vi "Bertta_v06_1.vi"() -> ()   [LabVIEW 2015]
uses:
  BERTTA.dll
panel:
  in  "Tab Control":T1(tab)
  in  "Description":string
  in  "Project name":string
  in  "User (initials)":string
  out "Tr":dbl
  out "Tj":dbl
  out "Numeric 2":dbl
  out "Numeric 3":dbl
  out "Numeric":dbl
  out "Mettler 5":dynamicdata(graph)
  out "Temp":dynamicdata(graph)
  out "Mettler":dynamicdata(graph)
  in  "Balances":bool[](array[boolean])
  out "Waveform Chart 3":dynamicdata(graph)
  out "Table":string[][](table)
  in  "Headers":string[](array[string])
  in  "?":bool
  in  "Seq":dbl[][](array[numeric])=[[20.0, 60.0, 40.0], [60.0, 40.0, 20.0], [100.0, 100.0, 100.0]]
  out "Elapsed":i32
  out "Step":i32
  out "Sp":dbl
  out "T":dbl
  out "Tinit":dbl
  out "Tset":dbl
  out "Time constant":dbl
  out "Sp - Tset":i32
  out "Change":i32
  out "Waveform Chart":dynamicdata(graph)
  in  "Tbypass":dbl=33.0
  in  "Tfail":dbl=22.0
  in  "err":i32
  in  "PAUSE":bool
  out "Waveform Chart 2":dynamicdata(graph)
  out "Rate (g/s)":dbl
  out "Time (s)":dbl
  out "Target (g)":dbl
  in  "Seq 2":dbl[][](array[numeric])=[[20.0, 60.0, 40.0], [60.0, 40.0, 20.0], [100.0, 100.0, 100.0]]
  out "Weight (1)":dbl
  out "target reached":i32
  out "x/y":dbl
  out "bal_previous":i32
  out "Step":i32
  in  "?":bool
  in  "Bypass ramp":dbl
  in  "bypass 2":bool
  out "DAQ assistant (4-20 mA)":dbl
  out "Step":i32
  out "bal_previous":i32
  out "x/y":dbl
  out "target reached":i32
  out "Waveform Chart 5":dynamicdata(graph)
  out "Weight (2)":dbl
  out "Rate (g/s)":dbl
  out "Time (s)":dbl
  out "Target (g)":dbl
  in  "Seq 3":dbl[][](array[numeric])=[[20.0, 60.0, 40.0], [60.0, 40.0, 20.0], [100.0, 100.0, 100.0]]
  in  "Boolean":bool
  in  "Bypass ramp":dbl
  in  "bypass":bool
  out "RS232 to Ismatec":dbl
  in  "Boolean 2":bool
  out "Step":i32
  out "bal_previous":i32
  out "x/y":dbl
  out "target reached":i32
  out "Waveform Chart 6":dynamicdata(graph)
  out "Weight (3)":dbl
  out "Rate (g/s)":dbl
  out "Time (s)":dbl
  out "Target (g)":dbl
  in  "Seq 4":dbl[][](array[numeric])=[[20.0, 60.0, 40.0], [60.0, 40.0, 20.0], [100.0, 100.0, 100.0]]
  in  "Boolean 3":bool
  out "Step":i32
  out "bal_previous":i32
  out "x/y":dbl
  out "target reached":i32
  out "Waveform Chart 7":dynamicdata(graph)
  out "Weight (4)":dbl
  out "Rate (g/s)":dbl
  out "Time (s)":dbl
  out "Target (g)":dbl
  in  "Seq 5":dbl[][](array[numeric])=[[20.0, 60.0, 40.0], [60.0, 40.0, 20.0], [100.0, 100.0, 100.0]]
  out "RPM":dbl
  out "Waveform Chart 4":dynamicdata(graph)
  in  "Set RPM":dbl(slide) scale=0.0..500.0
  out "Torque":dbl
  in  "?":T2(tab)
  in  "Device port":dbl=1.0
  out "Debug msg":dbl
  in  "Device port":dbl=8.0
  in  "Device port":i32=2
  in  "Device port 2":i32=6
  in  "Device port 3":i32=7
  in  "Device port 4":i32=10
  # "1"
  # "2"
  # "3"
  # "4"
  # "Step 1"
  # "Step 2"
  # "Step 3"
  # "Step 4"
  # "Step 1"
  # "Step 2"
  # "Step 3"
  # "Step 4"
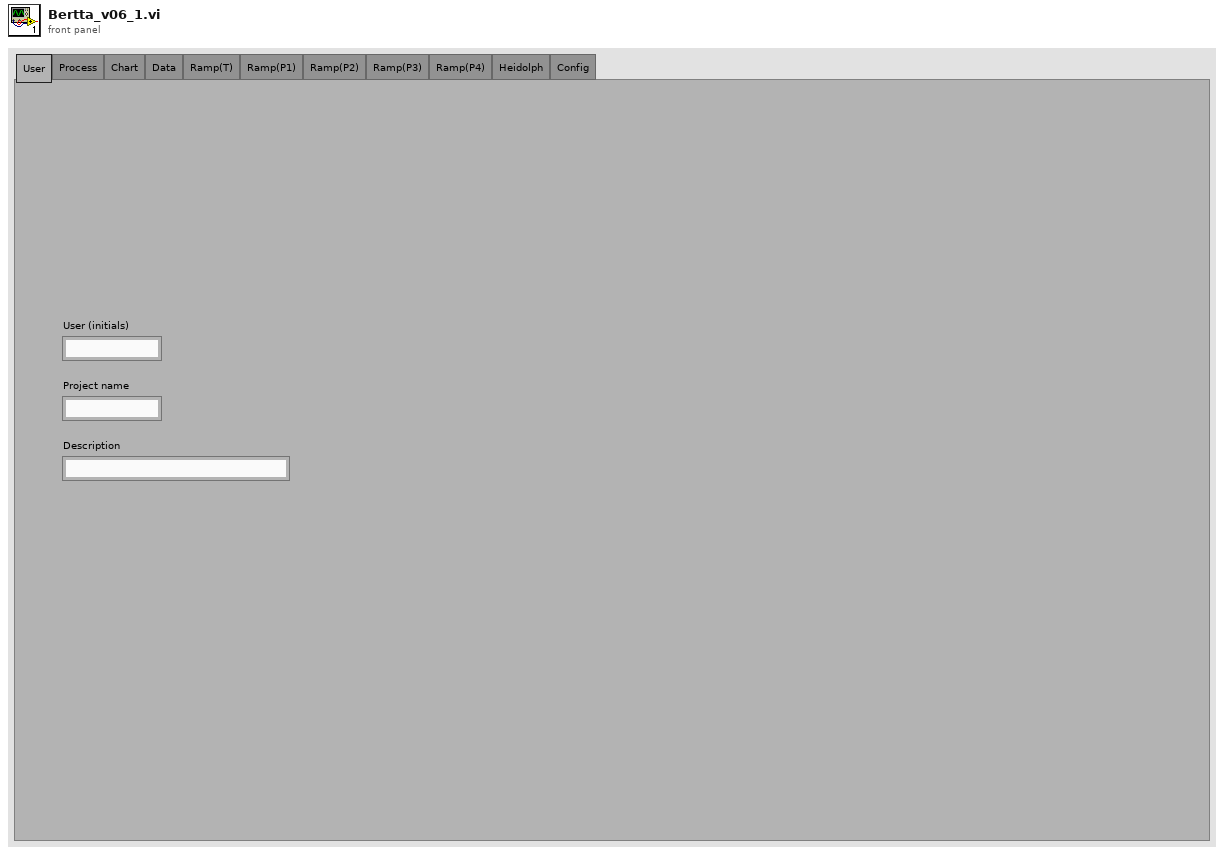
[diagram p1: front panel]
types:
  T1 = enum32{"User", "Process", "Chart", "Data", "Ramp(T)", "Ramp(P1)", "Ramp(P2)", "Ramp(P3)", "Ramp(P4)", "Heidolph", "Config"}
  T2 = enum32{"DB / File", "Lauda", "Heidolph", "Mettler 1", "Mettler 2", "Mettler 3", "Ismatec 1"}
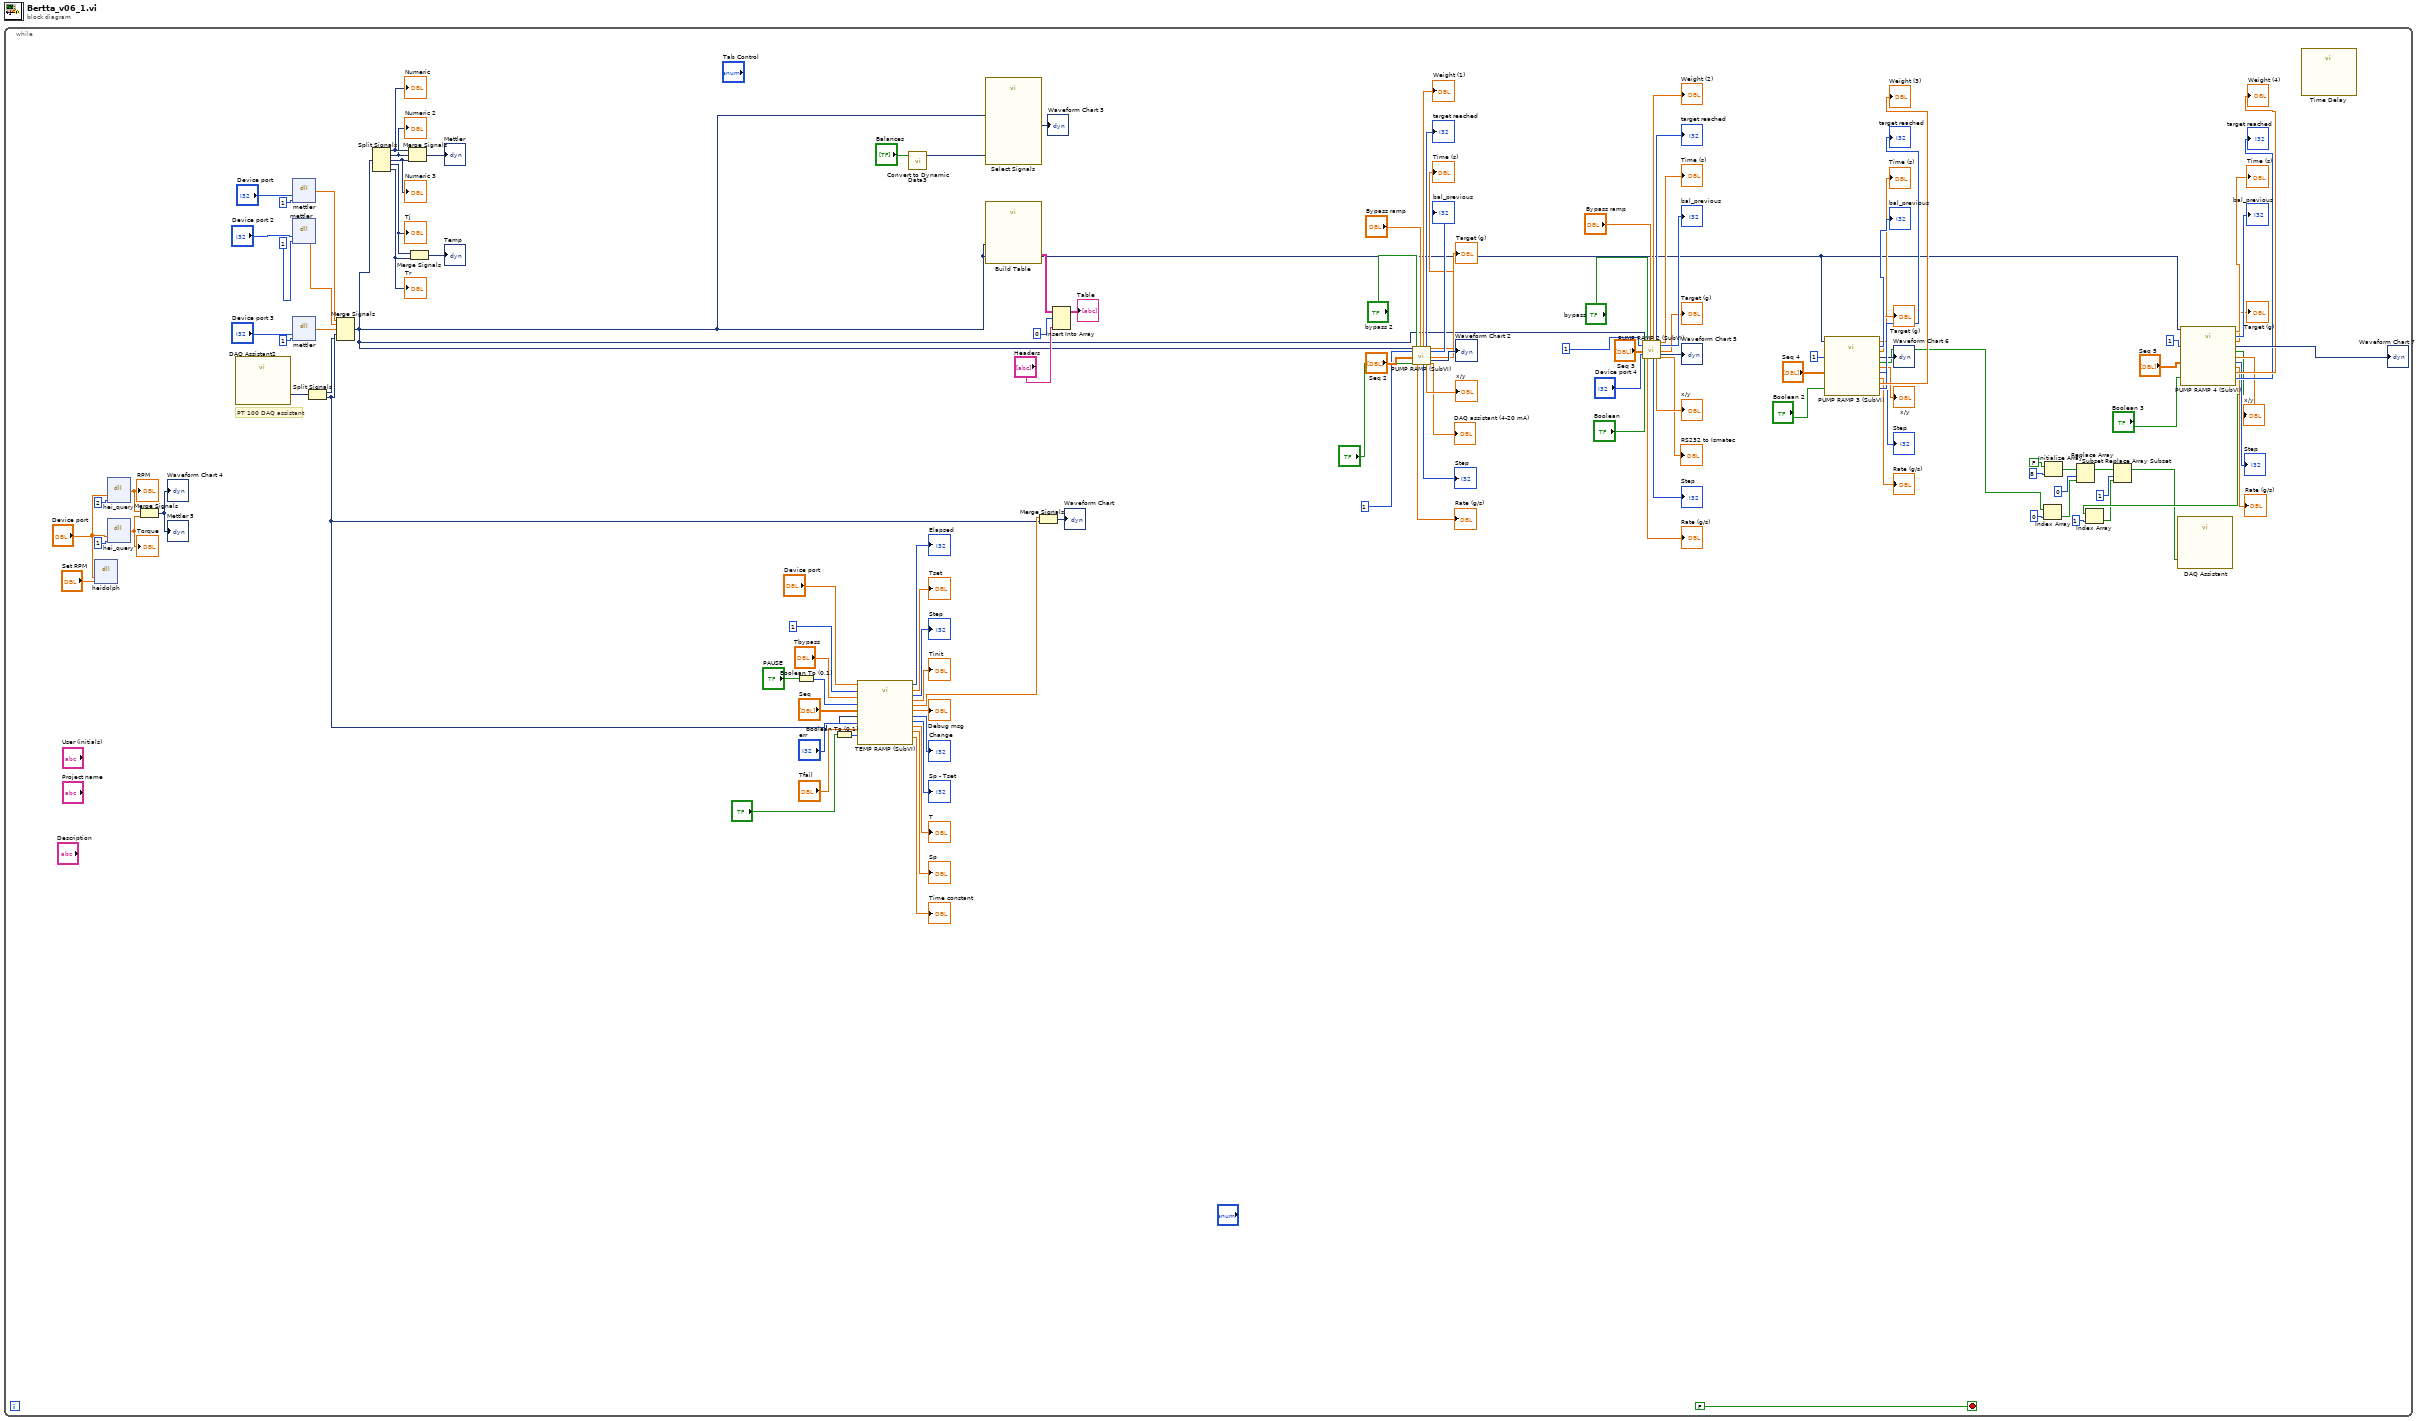
[diagram p0: block diagram]
diagram:
  n1 = while {
    stop <- FALSE stop-if-true
    # "PT 100 DAQ assistant"
    n2 = dll-call lib="C:/Users/xlaraser/Documents/Visual Studio 2017/Projects/Bertta/BERTTA/Debug/BERTTA.dll" fn="heidolph"("port"="Device port", "speed"="Set RPM") -> ()  [unwired: 6 in, 2 out]
    n3 = dll-call lib="C:/Users/xlaraser/Documents/Visual Studio 2017/Projects/Bertta/BERTTA/Debug/BERTTA.dll" fn="hei_query"("port"="Device port", "q"=2) -> ("return type"=w108:dbl)  [unwired: 5 in, 2 out]
    "RPM" <- w108
    n4 = dll-call lib="C:/Users/xlaraser/Documents/Visual Studio 2017/Projects/Bertta/BERTTA/Debug/BERTTA.dll" fn="hei_query"("port"="Device port", "q"=1) -> ("return type"=w107:dbl)  [unwired: 5 in, 2 out]
    "Torque" <- w107
    n5 = Merge Signals(w108, w107) -> (→"Waveform Chart 4" →"Mettler 5":dynamicdata)
    n6 = call "DAQ Assistant2"() -> ("data"=w11:dynamicdata)  [unwired: 17 in, 2 out]
    n7 = dll-call lib="C:/Users/xlaraser/Documents/Visual Studio 2017/Projects/Bertta/BERTTA/Debug/BERTTA.dll" fn="mettler"("port"="Device port", "msg"=1) -> ("return type"=w72:dbl)  [unwired: 5 in, 2 out]
    n8 = dll-call lib="C:/Users/xlaraser/Documents/Visual Studio 2017/Projects/Bertta/BERTTA/Debug/BERTTA.dll" fn="mettler"("port"="Device port 2", "msg"=1) -> ("return type"=w71:dbl)  [unwired: 5 in, 2 out]
    n9 = dll-call lib="C:/Users/xlaraser/Documents/Visual Studio 2017/Projects/Bertta/BERTTA/Debug/BERTTA.dll" fn="mettler"("port"="Device port 3", "msg"=1) -> ("return type"=w58:dbl)  [unwired: 5 in, 2 out]
    n10 = Split Signals(w11) -> (w10:dynamicdata, w37:dynamicdata)  [unwired: 2 in]
    n11 = Merge Signals(w72, w71, w58, w37, w10) -> (w9:dynamicdata)
    n12 = Split Signals(w9) -> (w5:dynamicdata, w3:dynamicdata, w2:dynamicdata, w8:dynamicdata, w6:dynamicdata)  [unwired: 5 in]
    "Numeric" <- w5
    "Numeric 2" <- w3
    "Numeric 3" <- w2
    "Tr" <- w6
    "Tj" <- w8
    n13 = Merge Signals(w5, w3, w2) -> (→"Mettler":dynamicdata)
    n14 = Merge Signals(w8, w6) -> (→"Temp":dynamicdata)
    n15 = Boolean To (0,1)(Boolean="PAUSE") -> (0, 1=w85:i16)
    n16 = Boolean To (0,1)(Boolean="?") -> (0, 1=w53:i16)
    n17 = call "TEMP RAMP (SubVI).vi"("Device port"="Device port", "Numeric"=i16 1, "Tbyp"="Tbypass", "Numeric 2"=w85, "Seq"="Seq", "data"=w37, "bypass"=w53, "err"="err", "Tfail"="Tfail") -> ("Sp - Tset"=→"Sp - Tset":i32, "T"=→"T":dbl, "Sp"=→"Sp":dbl, "Change"=→"Change":i32, "tr"=→"Time constant":dbl, "Debug msg"=→"Debug msg":dbl, "Elapsed"=→"Elapsed":i32, "Tset"=→"Tset":dbl, "Step"=→"Step":i32, "Tinit"=→"Tinit":dbl, "return type"=w113:dbl)
    n18 = call "Convert to Dynamic Data3"("Array"="Balances") -> ("Dynamic Data Type"=w116:dynamicdata)  [unwired: 3 in]
    n19 = call "Select Signals"("Selector Input"=w116, "Signals"=w9) -> ("Signal Out"=→"Waveform Chart 3":dynamicdata)  [unwired: 8 in, 1 out]
    n20 = call "Build Table"("Signals"=w9) -> ("Table"=w119:string[][])  [unwired: 4 in, 6 out]
    n21 = Merge Signals(w113, w37) -> (→"Waveform Chart":dynamicdata)
    n22 = Insert Into Array(array=w119, index (row)=0, new element="Headers") -> (→"Table":string[][])  [unwired: 1 in]
    n23 = call "PUMP RAMP (SubVI).vi"("Dynamic Data"=w9, "Numeric"=i16 1, "Seq in"="Seq 2", 5:"?", "bypass"="bypass 2", "bypass RPM"="Bypass ramp") -> ("Rate (g/s)"=→"Rate (g/s)":dbl, "Weight (S1)"=→"Weight (1)":dbl, "Step 2"=→"Step":i32, "target reached"=→"target reached":i32, "x/y"=→"x/y":dbl, "Time (s)"=→"Time (s)":dbl, "bal_previous"=→"bal_previous":i32, "Target (g)"=→"Target (g)":dbl, "Waveform Chart 2"=→"Waveform Chart 2":dynamicdata, "DAQ assistant (4-20 mA)"=→"DAQ assistant (4-20 mA)":dbl)  [unwired: 4 in]
    n24 = call "PUMP RAMP 2 (SubVI).vi"("Dynamic Data"=w9, "Numeric"=i16 1, "Seq in"="Seq 3", "Device port"="Device port 4", "enable"="Boolean", "bypass"="bypass", "bypass RPM"="Bypass ramp") -> ("Rate (g/s)"=→"Rate (g/s)":dbl, "Weight (S1)"=→"Weight (2)":dbl, "Step 2"=→"Step":i32, "target reached"=→"target reached":i32, "x/y"=→"x/y":dbl, "Time (s)"=→"Time (s)":dbl, "bal_previous"=→"bal_previous":i32, "Target (g)"=→"Target (g)":dbl, "Waveform Chart 2"=→"Waveform Chart 5":dynamicdata, "RS232 to Ismatec"=→"RS232 to Ismatec":dbl)  [unwired: 3 in]
    n25 = call "PUMP RAMP 3 (SubVI).vi"("Dynamic Data"=w9, "Numeric"=i16 1, "Seq in"="Seq 4", "Boolean"="Boolean 2") -> ("Weight (S1)"=→"Weight (3)":dbl, "target reached"=→"target reached":i32, "Time (s)"=→"Time (s)":dbl, "bal_previous"=→"bal_previous":i32, "Target (g)"=→"Target (g)":dbl, "Waveform Chart 2"=→"Waveform Chart 6":dynamicdata, "Rate (g/s)"=→"Rate (g/s)":dbl, "Step 2"=→"Step":i32, "x/y"=→"x/y":dbl, "DAQ assistant (PAM i/o)"=w22:bool[])  [unwired: 2 in]
    n26 = Index Array(array=w22, index=0) -> (element=w16:bool)
    n27 = Initialize Array(FALSE ("element"), 8 ("dimension size")) -> (w18:bool[])
    n28 = Replace Array Subset(array=w18, new element=w16, index=0) -> (w12:bool[])
    n29 = call "PUMP RAMP 4 (SubVI).vi"("Dynamic Data"=w9, "Numeric"=i16 1, "Seq in"="Seq 5", "Boolean"="Boolean 3") -> ("Weight (S1)"=→"Weight (4)":dbl, "target reached"=→"target reached":i32, "Time (s)"=→"Time (s)":dbl, "bal_previous"=→"bal_previous":i32, "Target (g)"=→"Target (g)":dbl, "Waveform Chart 2"=→"Waveform Chart 7":dynamicdata, "Rate (g/s)"=→"Rate (g/s)":dbl, "Step 2"=→"Step":i32, "x/y"=→"x/y":dbl, "DAQ assistant (PAM i/o)"=w19:bool[])  [unwired: 2 in]
    n30 = Index Array(array=w19, index=1) -> (element=w14:bool)
    n31 = Replace Array Subset(array=w12, new element=w14, index=1) -> (w15:bool[])
    n32 = call "DAQ Assistant"("data"=w15) -> ()  [unwired: 17 in, 2 out]
    n33 = call "Time Delay"() -> ()  [unwired: 11 in, 1 out]
  }
